vi "Scan action control.vi"(0 "Index":dbl, 1 "OSC Configuration":T2(array[cluster])=[{"Signal Type"=enum."Sawtooth Wave", "DC"=0.00035, "Amplitude"=0.002, "frequency"=0.4, "Phase"=180.0}, {"Signal Type"=enum."Sine Wave", "DC"=0.0, "Amplitude"=0.0, "frequency"=1.0, "Phase"=0.0}, {"Signal Type"=enum."Sine Wave", "DC"=0.0, "Amplitude"=0.0, "frequency"=1.0, "Phase"=0.0}, {"Signal Type"=enum."Sine Wave", "DC"=0.0, "Amplitude"=0.0, "frequency"=1.0, "Phase"=0.0}] {"frequency" format="%0.2p"; "Amplitude" format="%0.2p"; "DC" format="%.2p"}, 2 "Scan control":u16(ring)=5 items=["OFF", "Vsg1", "Vsg2", "Vsgw", "Vbg", "Field", "Temp"], 3 "Scan Parameters":T1={"DAQ Channel"=3, "Label"="\nappliedFiled=", "Scaled low"=-0.060000000000000005, "Scaled high"=0.14, "Start"=-1000.0, "End"=-6000.0, "Step"=1000.0, "Scale?"=FALSE} {"Step" format="%#_6p"; "End" format="%#_6p"; "Start" format="%#_6p"; "Scaled high" format="%#_6p"; "Scaled low" format="%#_6p"}, 4 "Comments":string="SA02704G.20140508\n2mVac+350uVdc\nBackgate=-6.7V\n\nsweep Vsg -0.25V to 0.25V, 0.0005V steps\nsweep Field -1000oe to -6000oe\n") -> (5 "Comments out":string="SA02704G.20140508\n2mVac+350uVdc\nBackgate=-6.7V\n\nsweep Vsg -0.25V to 0.25V, 0.0005V steps\nsweep Field -1000oe to -6000oe\n\nappliedFiled= -1000.000000", 6 "OSC Configuration out":T2(array[cluster])=[{"Signal Type"=enum."Sawtooth Wave", "DC"=0.00035, "Amplitude"=0.002, "frequency"=0.4, "Phase"=180.0}, {"Signal Type"=enum."Sine Wave", "DC"=0.0, "Amplitude"=0.0, "frequency"=1.0, "Phase"=0.0}, {"Signal Type"=enum."Sine Wave", "DC"=0.0, "Amplitude"=0.0, "frequency"=1.0, "Phase"=0.0}, {"Signal Type"=enum."Sine Wave", "DC"=0.0, "Amplitude"=0.0, "frequency"=1.0, "Phase"=0.0}] {"frequency" format="%0.2p"; "Amplitude" format="%0.2p"; "DC" format="%.2p"}, 7 "Stop?":bool)   [LabVIEW 2013]
panel:
  in  "Rate (K/min)":dbl=5.0
  in  "Rate (Oe/s)":i32=50
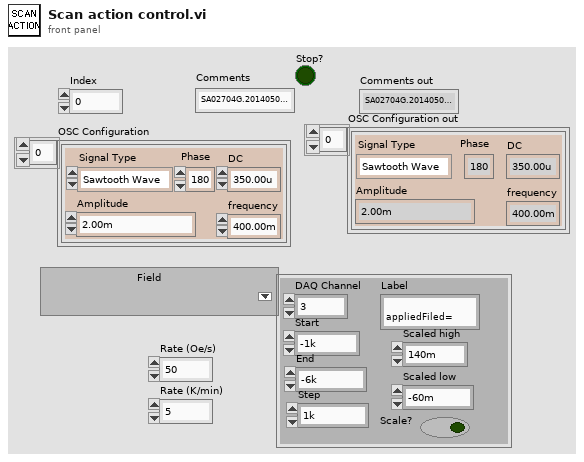
[diagram p1: front panel]
types:
  T1 = cluster{"DAQ Channel":i32, "Label":string, "Scaled low":dbl, "Scaled high":dbl, "Start":dbl, "End":dbl, "Step":dbl, "Scale?":bool}
  T2 = cluster{"Signal Type":enum16{"Sine Wave", "Triangle Wave", "Square Wave", "Sawtooth Wave"}, "DC":dbl, "Amplitude":dbl, "frequency":dbl, "Phase":dbl}[]
  T3 = cluster{"Signal Type":enum16{"Sine Wave", "Triangle Wave", "Square Wave", "Sawtooth Wave"}, "DC":dbl, "Amplitude":dbl, "frequency":dbl, "Phase":dbl}
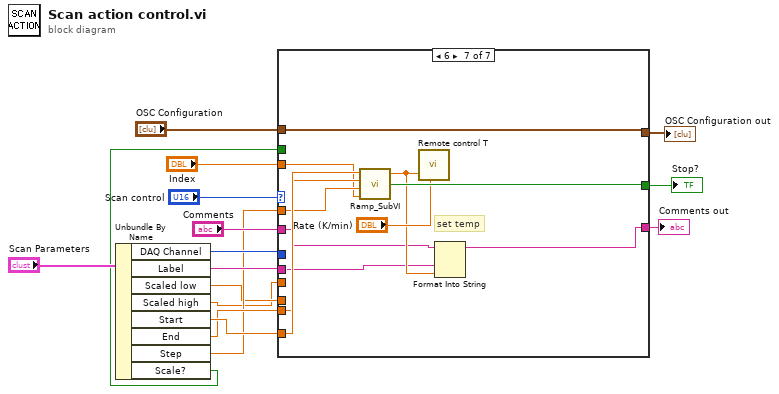
[diagram p0: block diagram]
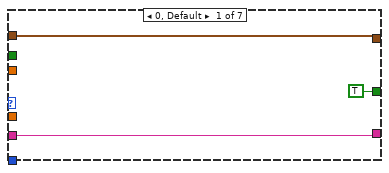
[diagram p2: hidden frame]
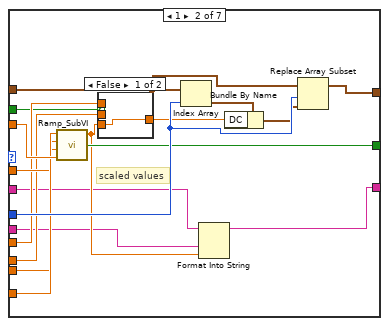
[diagram p3: hidden frame]
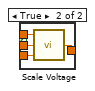
[diagram p4: hidden frame]
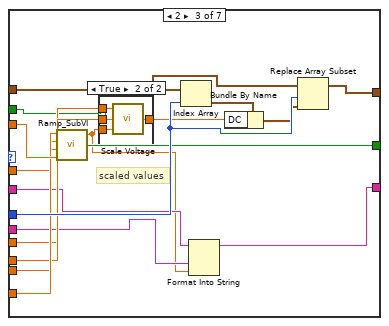
[diagram p5: hidden frame]
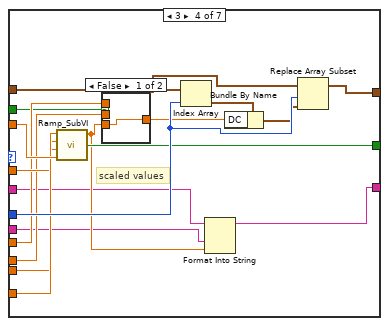
[diagram p7: hidden frame]
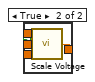
[diagram p8: hidden frame]
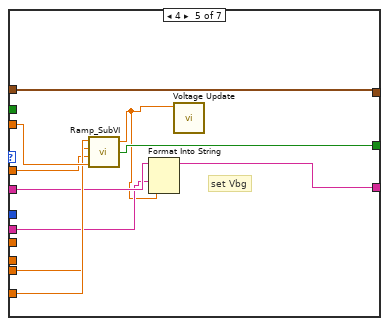
[diagram p9: hidden frame]
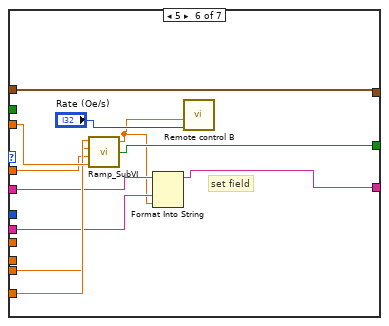
[diagram p10: hidden frame]
diagram:
  n1 = Unbundle By Name("Scan Parameters") -> ("DAQ Channel"=w14:i32, "Label"=w12:string, "Scaled low"=w3:dbl, "Scaled high"=w2:dbl, "Start"=w7:dbl, "End"=w6:dbl, "Step"=w5:dbl, "Scale?"=w1:bool)
  n2 = case shown="6" "Scan control" {
    tunnel: "OSC Configuration" -> [w19 w36 w59 w82 w98 w109 w120]
    tunnel: w14 -> [_ w35 w58 w81 _ _ _]
    tunnel: [w19 w33 w56 w79 w98 w109 w120] -> w11
    tunnel: "Comments" -> [w18 w21 w46 w67 w92 w102 w111]
    tunnel: [w18 w22 w43 w68 w89 w99 w110] -> w10
    tunnel: w12 -> [_ w20 w45 w66 w91 w101 w112]
    tunnel: "Index" -> [_ w32 w55 w78 w97 w108 w116]
    tunnel: w7 -> [_ w31 w54 w77 w96 w107 w119]
    tunnel: w6 -> [_ w30 w53 w76 w95 w106 w118]
    tunnel: w5 -> [_ w29 w52 w75 w94 w105 w117]
    tunnel: [TRUE ("Stop?") w28 w51 w74 w93 w104 w115] -> w4
    tunnel: w3 -> [_ w26 w50 w72 _ _ _]
    tunnel: w2 -> [_ w27 w49 w73 _ _ _]
    tunnel: w1 -> [_ w24 w47 w70 _ _ _]
    frame 0, Default {
    }
    frame 1 {
      # "scaled values"
      n3 = call <userlib>:"Ramp_SubVI.vi"("index"=w32, "step"=w29, "end"=w30, "start"=w31) -> ("Stop?"=w28:bool, "Numeric"=w23:dbl)  [unwired: 1 in]
      n4 = case shown="False" w24 {
        tunnel: w27 -> [_ w42]
        tunnel: w26 -> [_ w41]
        tunnel: w23 -> [w38 w40]
        tunnel: [w38 w39] -> w25
        frame False {
        }
        frame True {
          n5 = call "Scale Voltage.vi"("Scale factor"=w40, "Breakdown Low"=w41, "Breakdown High"=w42) -> ("Real Voltage"=w39:dbl)
        }
      }
      n6 = Index Array(array=w36, index=w35) -> (element=w37:T3)
      n7 = Format Into String(initial string=w21, w20, w23) -> (resulting string=w22:string)  [unwired: 2 in, 1 out]
      n8 = Bundle By Name(cluster=w37, "DC"=w25) -> (w34:T3)
      n9 = Replace Array Subset(array=w36, new element=w34, index=w35) -> (w33:T2)
    }
    frame 2 {
      # "scaled values"
      n10 = call <userlib>:"Ramp_SubVI.vi"("index"=w55, "step"=w52, "end"=w53, "start"=w54) -> ("Stop?"=w51:bool, "Numeric"=w44:dbl)  [unwired: 1 in]
      n11 = case shown="True" w47 {
        tunnel: w50 -> [_ w65]
        tunnel: w49 -> [_ w64]
        tunnel: w44 -> [w61 w63]
        tunnel: [w61 w62] -> w48
        frame False {
        }
        frame True {
          n12 = call "Scale Voltage.vi"("Scale factor"=w63, "Breakdown Low"=w65, "Breakdown High"=w64) -> ("Real Voltage"=w62:dbl)
        }
      }
      n13 = Index Array(array=w59, index=w58) -> (element=w60:T3)
      n14 = Format Into String(initial string=w46, w45, w44) -> (resulting string=w43:string)  [unwired: 2 in, 1 out]
      n15 = Bundle By Name(cluster=w60, "DC"=w48) -> (w57:T3)
      n16 = Replace Array Subset(array=w59, new element=w57, index=w58) -> (w56:T2)
    }
    frame 3 {
      # "scaled values"
      n17 = call <userlib>:"Ramp_SubVI.vi"("index"=w78, "step"=w75, "end"=w76, "start"=w77) -> ("Stop?"=w74:bool, "Numeric"=w69:dbl)  [unwired: 1 in]
      n18 = case shown="False" w70 {
        tunnel: w69 -> [w84 w88]
        tunnel: w73 -> [_ w87]
        tunnel: w72 -> [_ w86]
        tunnel: [w84 w85] -> w71
        frame False {
        }
        frame True {
          n19 = call "Scale Voltage.vi"("Scale factor"=w88, "Breakdown Low"=w86, "Breakdown High"=w87) -> ("Real Voltage"=w85:dbl)
        }
      }
      n20 = Index Array(array=w82, index=w81) -> (element=w83:T3)
      n21 = Format Into String(initial string=w67, w66, w69) -> (resulting string=w68:string)  [unwired: 2 in, 1 out]
      n22 = Bundle By Name(cluster=w83, "DC"=w71) -> (w80:T3)
      n23 = Replace Array Subset(array=w82, new element=w80, index=w81) -> (w79:T2)
    }
    frame 4 {
      # "set Vbg"
      n24 = call <userlib>:"Ramp_SubVI.vi"("index"=w97, "step"=w94, "end"=w95, "start"=w96) -> ("Stop?"=w93:bool, "Numeric"=w90:dbl)  [unwired: 1 in]
      n25 = Format Into String(initial string=w92, w91, w90) -> (resulting string=w89:string)  [unwired: 2 in, 1 out]
      n26 = call "Voltage Update.vi"("Voltage Output"=w90) -> ()  [unwired: 8 in]
    }
    frame 5 {
      # "set field"
      n27 = call <userlib>:"Ramp_SubVI.vi"("index"=w108, "step"=w105, "end"=w106, "start"=w107) -> ("Stop?"=w104:bool, "Numeric"=w100:dbl)  [unwired: 1 in]
      n28 = Format Into String(initial string=w102, w101, w100) -> (resulting string=w99:string)  [unwired: 2 in, 1 out]
      n29 = call "Remote control B.vi"("Rate (Oe/s)"="Rate (Oe/s)", "Field (Oe)"=w100) -> ()  [unwired: 7 in, 1 out]
    }
    frame 6 {
      # "set temp"
      n30 = call <userlib>:"Ramp_SubVI.vi"("index"=w116, "step"=w117, "end"=w118, "start"=w119) -> ("Stop?"=w115:bool, "Numeric"=w113:dbl)  [unwired: 1 in]
      n31 = call "Remote control T.vi"("Temperature (K)"=w113, "Rate (K/min)"="Rate (K/min)") -> ()  [unwired: 4 in]
      n32 = Format Into String(initial string=w111, w112, w113) -> (resulting string=w110:string)  [unwired: 2 in, 1 out]
    }
  }
  "OSC Configuration out" <- w11
  "Comments out" <- w10
  "Stop?" <- w4
